vi "Head_tester.vi"() -> ()   [LabVIEW 2017]
panel:
  out "head.orientation.yaw":dbl
  out "head.orientation.pitch":dbl
  out "head.orientation.roll":dbl
  in  "Pitch offset":dbl
  out "error out":errorcluster
  in  "stop":bool
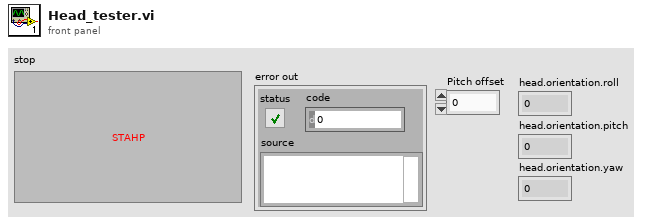
[diagram p1: front panel]
types:
  T1 = cluster{"head":cluster{"orientation":cluster{"roll":dbl, "pitch":dbl, "yaw":dbl}, "position":cluster{"x":dbl, "y":dbl, "z":dbl}}, "hands":cluster{"left":cluster{"position":cluster{"x":dbl, "y":dbl, "z":dbl}, "orientation":cluster{"roll":dbl, "pitch":dbl, "yaw":dbl}}, "right":cluster{"position":cluster{"x":dbl, "y":dbl, "z":dbl}, "orientation":cluster{"roll":dbl, "pitch":dbl, "yaw":dbl}}}, "buttons":cluster{"a":i32, "b":i32, "x":i32, "y":i32, "menu":i32, "leftTrig":dbl, "rightTrig":dbl, "leftGrip":dbl, "rightGrip":dbl, "left_jstick":cluster{"x":dbl, "y":dbl, "button":i32}, "right_jstick":cluster{"x":dbl, "y":dbl, "button":i32}}}
  T2 = typedef "Calibrated Oculus Data.ctl" = cluster{"head":cluster{"orientation":cluster{"roll":dbl, "pitch":dbl, "yaw":dbl}, "position":cluster{"x":dbl, "y":dbl, "z":dbl}}, "hands":cluster{"left":cluster{"position":cluster{"x":dbl, "y":dbl, "z":dbl}, "orientation":cluster{"roll":dbl, "pitch":dbl, "yaw":dbl}}, "right":cluster{"position":cluster{"x":dbl, "y":dbl, "z":dbl}, "orientation":cluster{"roll":dbl, "pitch":dbl, "yaw":dbl}}}, "buttons":cluster{"a":bool, "b":bool, "x":bool, "y":bool, "menu":bool, "leftTrig":dbl, "rightTrig":dbl, "leftGrip":dbl, "rightGrip":dbl, "left_jstick":cluster{"x":dbl, "y":dbl, "button":bool}, "right_jstick":cluster{"x":dbl, "y":dbl, "button":bool}}}
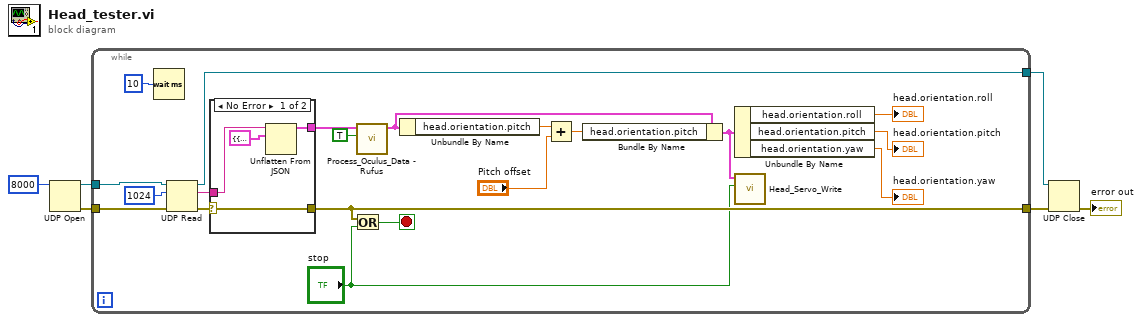
[diagram p0: block diagram]
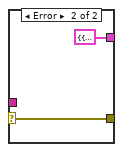
[diagram p2: hidden frame]
diagram:
  n1 = UDP Open(11:8000) -> (port=w4:refnum<k16>, 0:w5:errorcluster)  [unwired: 4 in, 1 out]
  n2 = while {
    tunnel: w5 -> [w26]
    tunnel: w4 -> [w25]
    tunnel: [w24] -> w3
    tunnel: [w18] -> w1
    stop <- w23 stop-if-true
    n3 = Wait (ms)(milliseconds to wait=u32 10) -> ()  [unwired: 1 out]
    n4 = UDP Read(connection ID=w25, max size (548)=1024, 8:w26) -> (data out=w21:string, error out=w22:errorcluster, 3:w24:refnum<k16>)  [unwired: 1 in, 2 out]
    n5 = case shown="No Error" w22 {
      selector: w22 -> [w29 w32]
      tunnel: [w29 w32] -> w18
      tunnel: w21 -> [w30 _]
      tunnel: [w28 T1 {"head"={"orientation"={"roll"=0.0, "pitch"=0.0, "yaw"=0.0}, "position"={"x"=0.0, "y"=0.0, "z"=0.0}}, "hands"={"left"={"position"={"x"=0.0, "y"=0.0, "z"=0.0}, "orientation"={"roll"=0.0, "pitch"=0.0, "yaw"=0.0}}, "right"={"position"={"x"=0.0, "y"=0.0, "z"=0.0}, "orientation"={"roll"=0.0, "pitch"=0.0, "yaw"=0.0}}}, "buttons"={"a"=0, "b"=0, "x"=0, "y"=0, "menu"=0, "leftTrig"=0.0, "rightTrig"=0.0, "leftGrip"=0.0, "rightGrip"=0.0, "left_jstick"={"x"=0.0, "y"=0.0, "button"=0}, "right_jstick"={"x"=0.0, "y"=0.0, "button"=0}}}] -> w17
      frame No Error {
        n6 = Unflatten From JSON(JSON string=w30, type and defaults=T1 {"head"={"orientation"={"roll"=0.0, "pitch"=0.0, "yaw"=0.0}, "position"={"x"=0.0, "y"=0.0, "z"=0.0}}, "hands"={"left"={"position"={"x"=0.0, "y"=0.0, "z"=0.0}, "orientation"={"roll"=0.0, "pitch"=0.0, "yaw"=0.0}}, "right"={"position"={"x"=0.0, "y"=0.0, "z"=0.0}, "orientation"={"roll"=0.0, "pitch"=0.0, "yaw"=0.0}}}, "buttons"={"a"=0, "b"=0, "x"=0, "y"=0, "menu"=0, "leftTrig"=0.0, "rightTrig"=0.0, "leftGrip"=0.0, "rightGrip"=0.0, "left_jstick"={"x"=0.0, "y"=0.0, "button"=0}, "right_jstick"={"x"=0.0, "y"=0.0, "button"=0}}}) -> (value=w28:T1)  [unwired: 5 in, 1 out]
      }
      frame Error {
      }
    }
    n7 = Or(x=w18, y="stop") -> (x .or. y?=w23:bool)
    n8 = call "Process_Oculus_Data - Rufus.vi"("Calibrated"=TRUE, "Raw Oculus Data"=w17) -> ("Calibrated Oculus Data"=w15:T2)  [unwired: 7 in, 2 out]
    n9 = Unbundle By Name(w15) -> ("head.orientation.pitch"=w14:dbl)
    n10 = Add(x=w14, y="Pitch offset") -> (x+y=w13:dbl)
    n11 = Bundle By Name(cluster=w15, "head.orientation.pitch"=w13) -> (w11:T2)
    n12 = Unbundle By Name(w11) -> ("head.orientation.roll"=→"head.orientation.roll":dbl, "head.orientation.pitch"=→"head.orientation.pitch":dbl, "head.orientation.yaw"=→"head.orientation.yaw":dbl)
    n13 = call "Head_Servo_Write.vi"("Stop"="stop", "Calibrated Oculus Data"=w11) -> ()  [unwired: 10 in]
  }
  n14 = UDP Close(connection ID=w3, 8:w1) -> (error out=→"error out":errorcluster)  [unwired: 1 out]
